vi "Change.vi"(0 "STEP in":refnum<class "STEP.lvclass">, 1 "Variables State":T3, 2 "SEQ":refnum<queue>, 3 "STEP State":T4, 4 "Current Sequence":T1, 5 "error in (no error)":errorcluster) -> (14 "STEP out":refnum<class "STEP.lvclass">, 15 "Variables State out":T3, 17 "STEP State out":T4, 19 "error out":errorcluster)   [LabVIEW 2014, in "SeqLoop.lvlib" / "STEP Classes.lvlib" / "STEP.lvclass"]
doc: "Gestiona el cambio de pasos en función del estado de la condición de avance, error y alarma."
uses:
  STEP.lvclass
  TypeDefs/STEP State.ctl
  APIs/Message Queue/Message Cluster.ctl
  TypeDefs/Variables State.ctl
  TypeDefs/Sequence.ctl
  TypeDefs/LogicParsedExpression.ctl
  STEP.lvclass/STEP.ctl
  APIs/Message Queue/Enqueue Message (Single).vi
  SeqLoop.lvlib
  APIs/Message Queue/WINFAS 2 Message Queue.lvlib
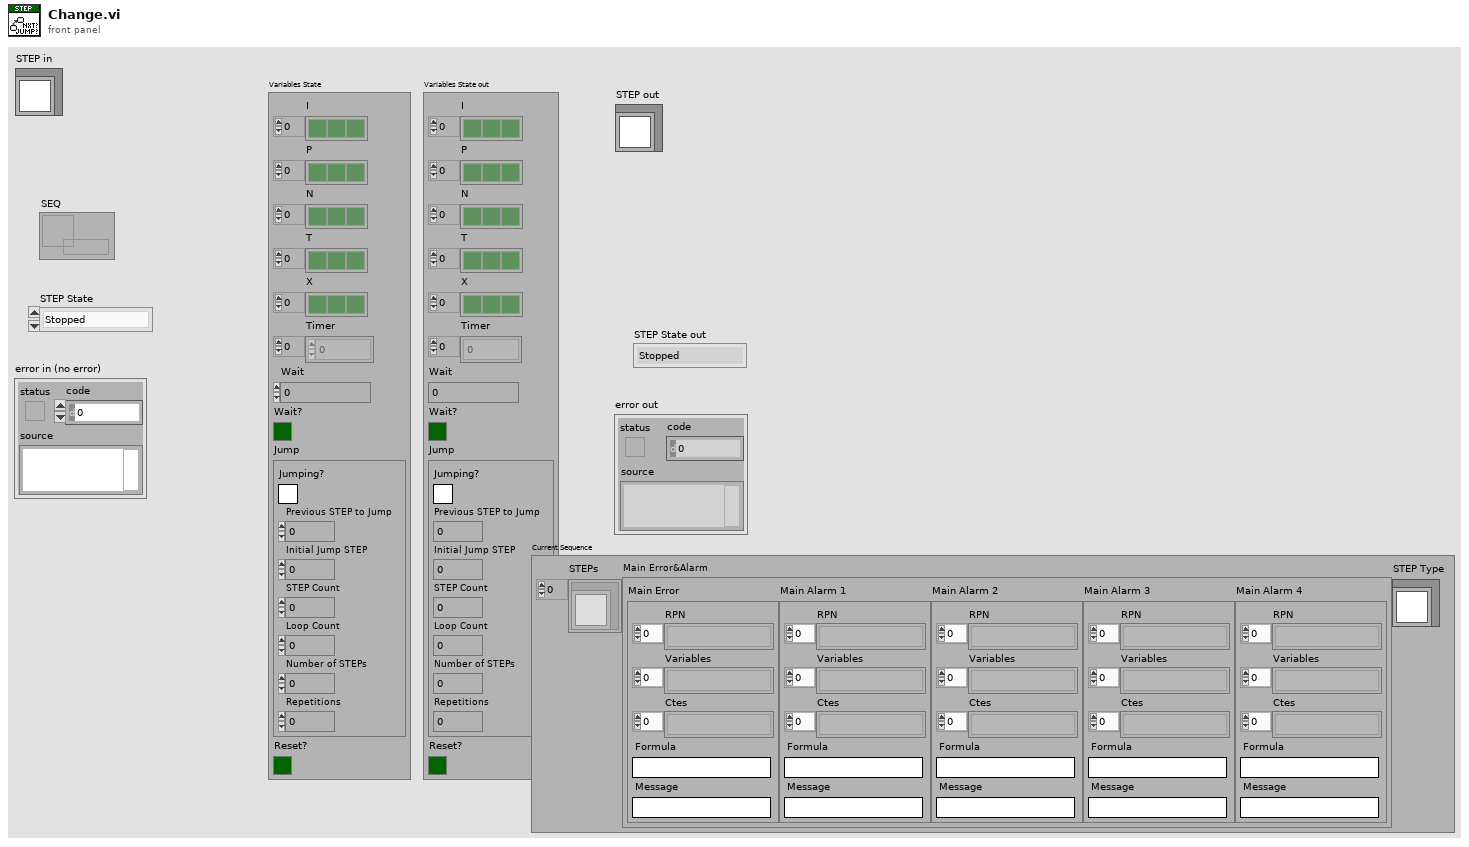
[diagram p1: front panel]
types:
  T1 = typedef "SeqLoop.lvlib/Sequence.ctl" = cluster{"STEPs":refnum<class "STEP.lvclass">[], "Main Error&Alarm":cluster{"Main Error":T2, "Main Alarm 1":T2, "Main Alarm 2":T2, "Main Alarm 3":T2, "Main Alarm 4":T2}, "STEP Type":refnum<class "STEP.lvclass">}
  T2 = typedef "SeqLoop.lvlib/LogicParsedExpression.ctl" = cluster{"RPN ":string[], "Variables":string[], "Ctes":string[], "Formula":string, "Message":string}
  T3 = typedef "SeqLoop.lvlib/Variables State.ctl" = cluster{"I":bool[], "P":bool[], "N":bool[], "T":bool[], "X":bool[], "Timer":u32[], "Wait":u32, "Wait?":bool, "Jump":cluster{"Jumping?":bool, "Previous STEP to Jump":u32, "Initial Jump STEP":u32, "STEP Count":u32, "Loop Count":u32, "Number of STEPs":u32, "Repetitions":u32}, "Reset?":bool}
  T4 = typedef "SeqLoop.lvlib/STEP State.ctl" = enum16{"Stopped", "First Call", "Idle...", "Advance OK", "Alarm", "Output Security", "Error"}
  T5 = cluster{"Jumping?":bool, "Previous STEP to Jump":u32, "Initial Jump STEP":u32, "STEP Count":u32, "Loop Count":u32, "Number of STEPs":u32, "Repetitions":u32}
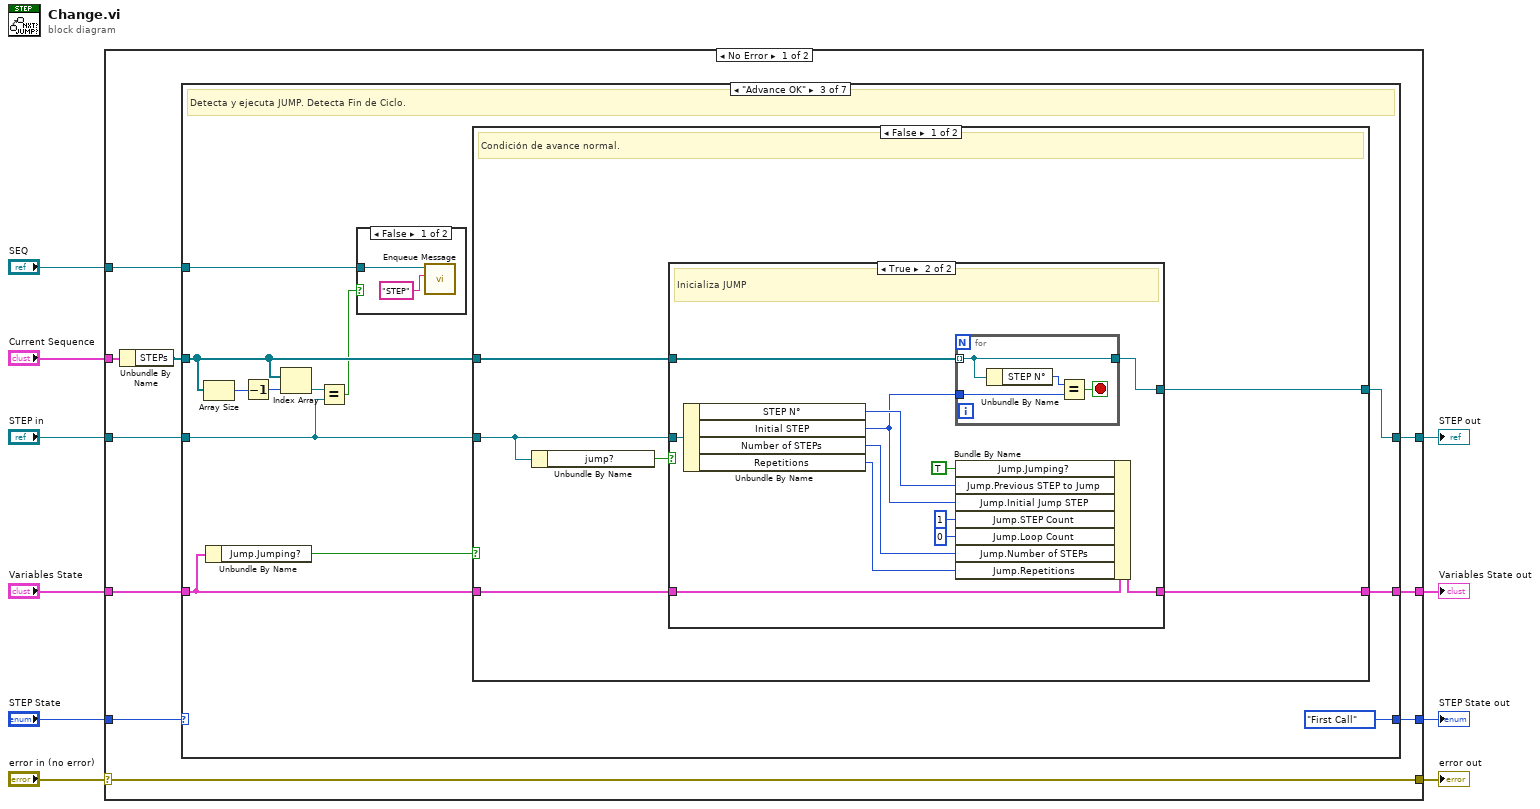
[diagram p0: block diagram]
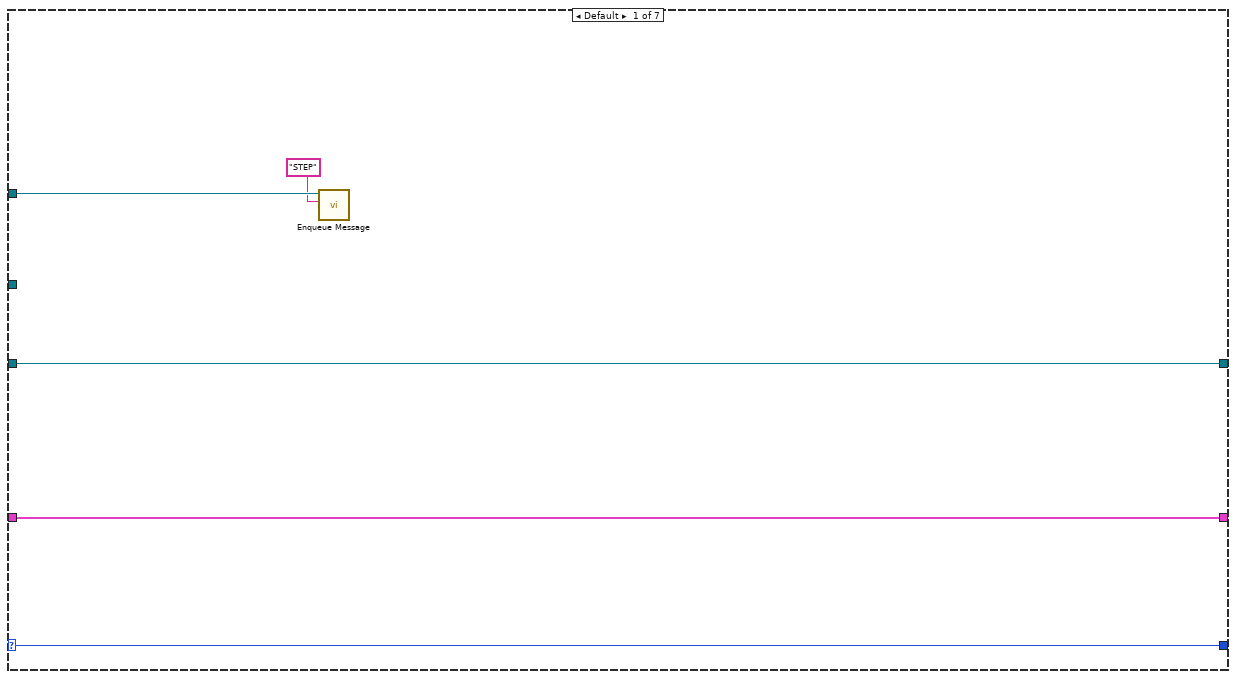
[diagram p2: hidden frame]
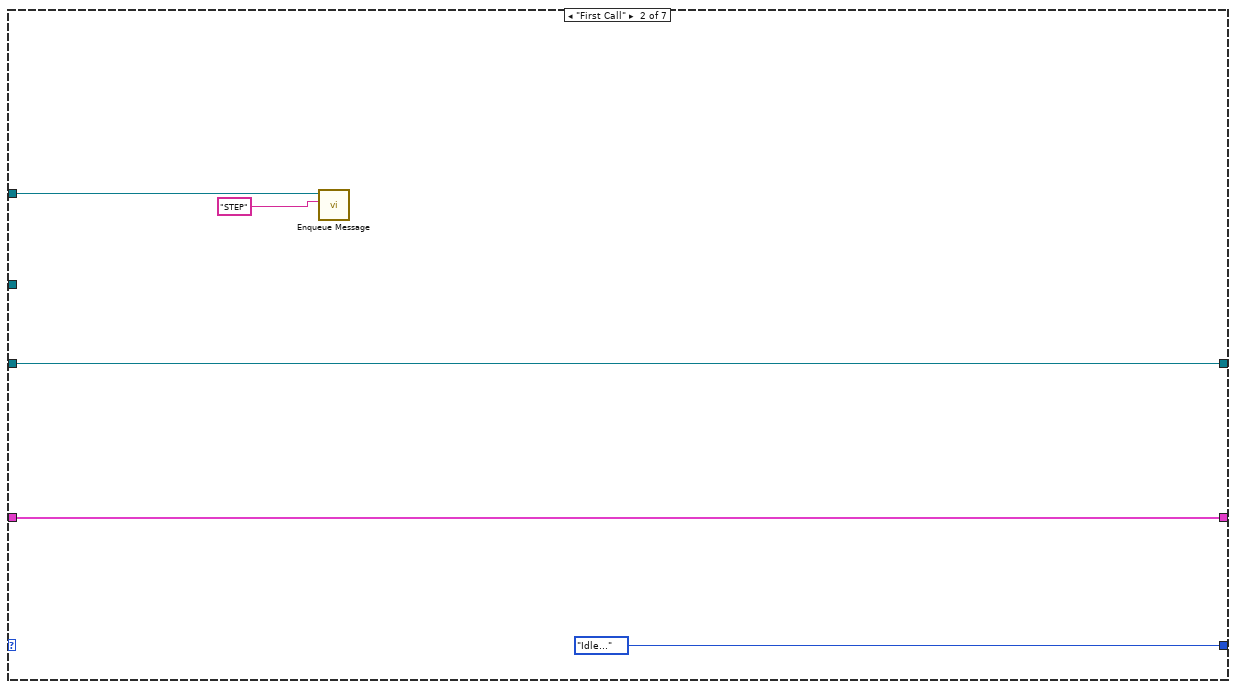
[diagram p3: hidden frame]
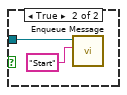
[diagram p4: hidden frame]
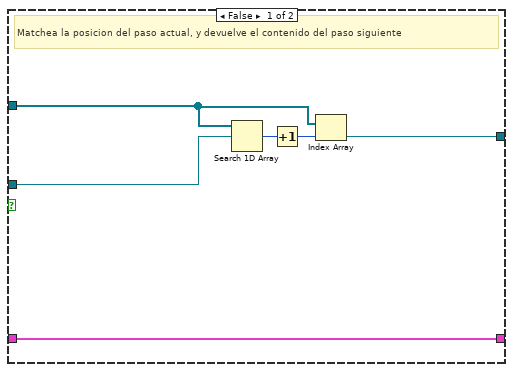
[diagram p5: hidden frame]
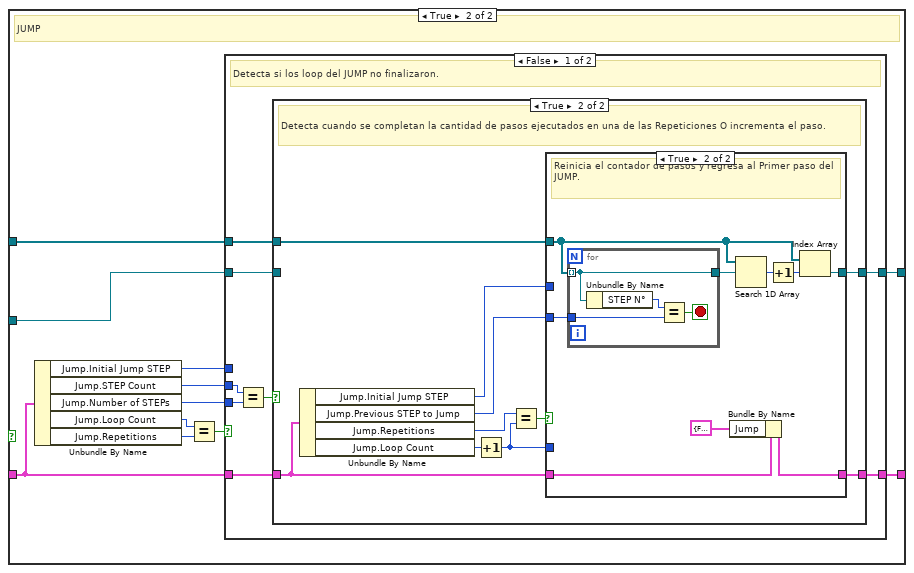
[diagram p6: hidden frame]
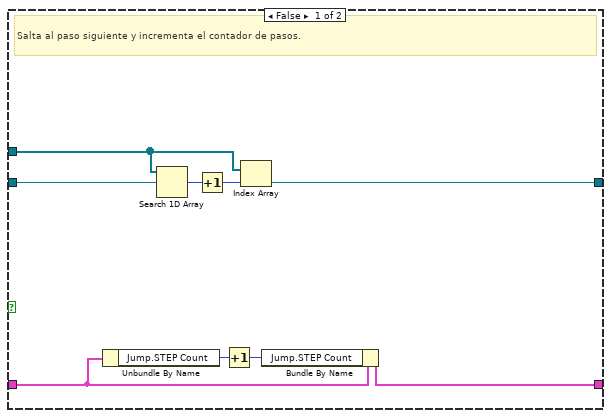
[diagram p7: hidden frame]
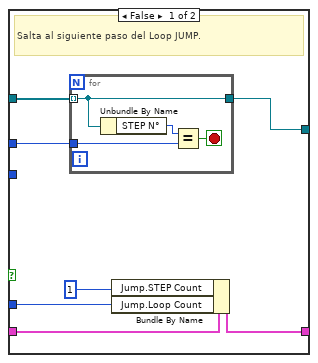
[diagram p8: hidden frame]
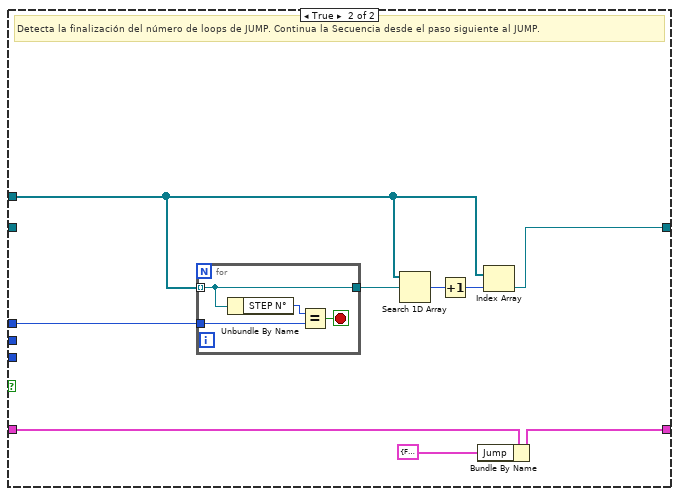
[diagram p9: hidden frame]
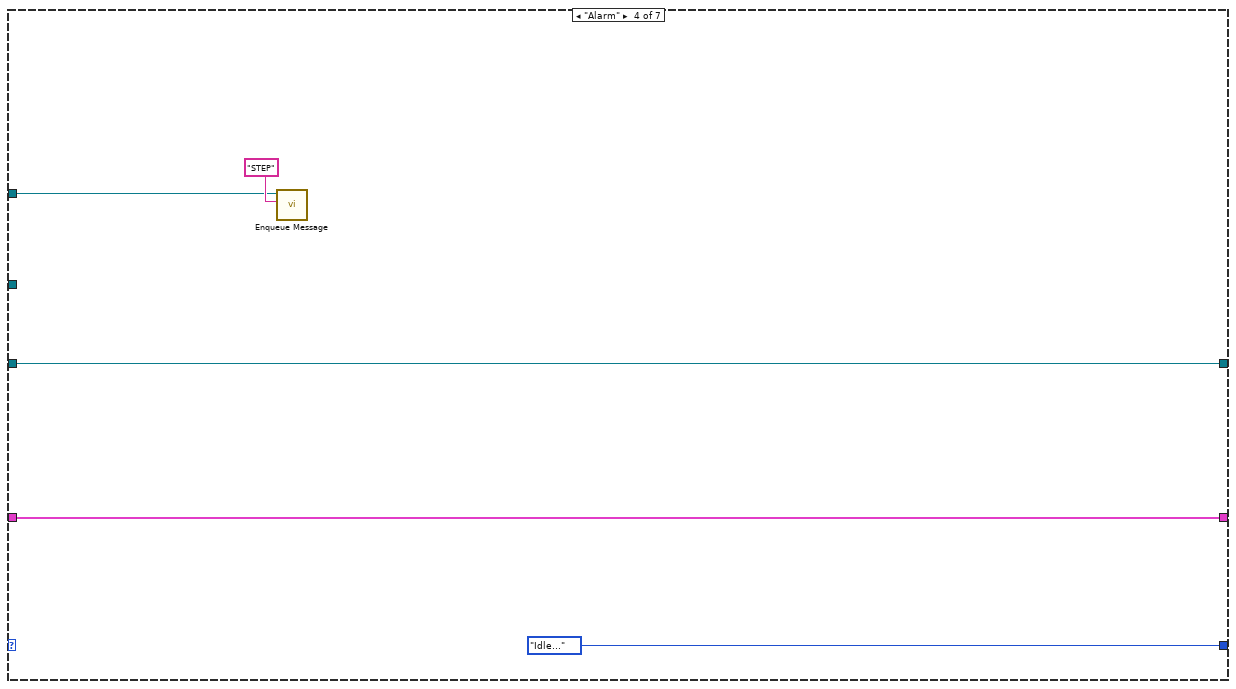
[diagram p10: hidden frame]
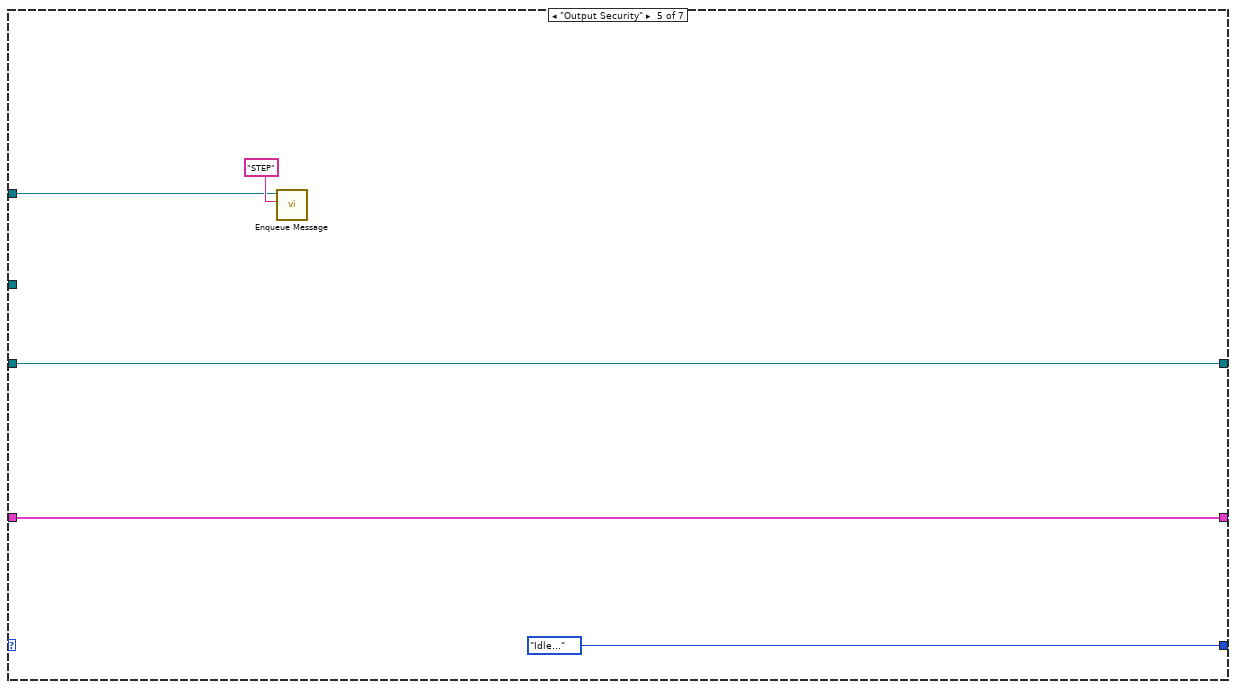
[diagram p11: hidden frame]
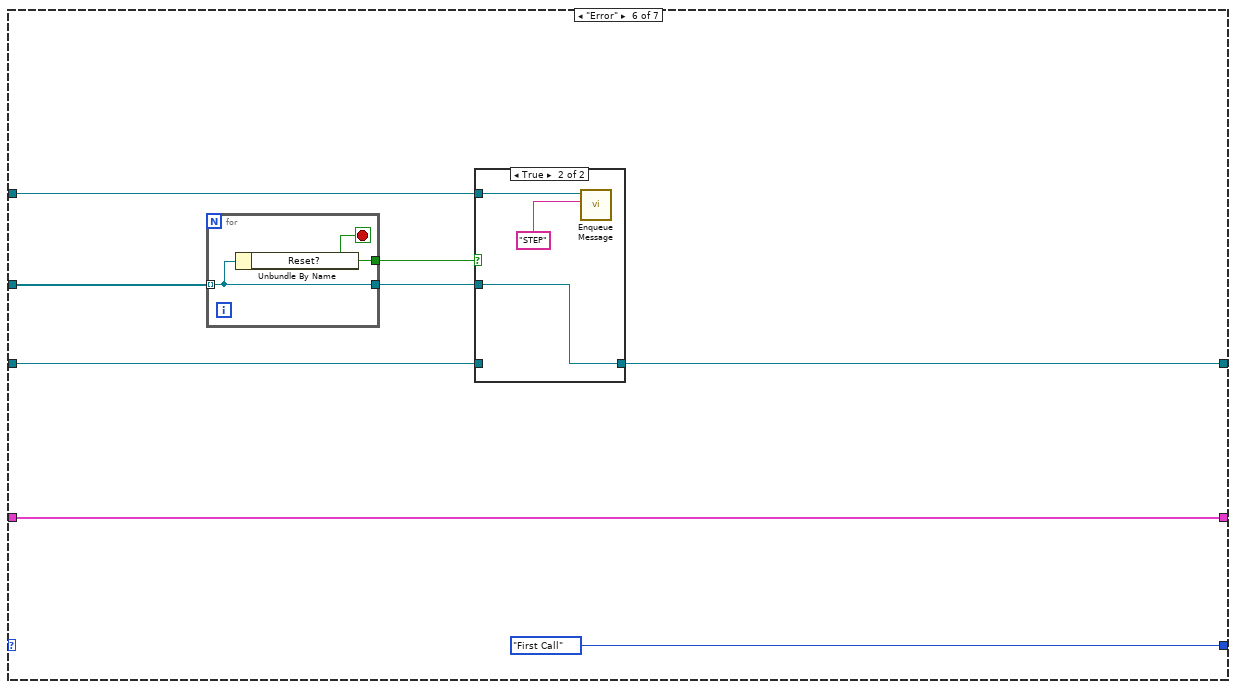
[diagram p12: hidden frame]
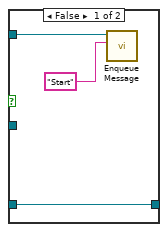
[diagram p13: hidden frame]
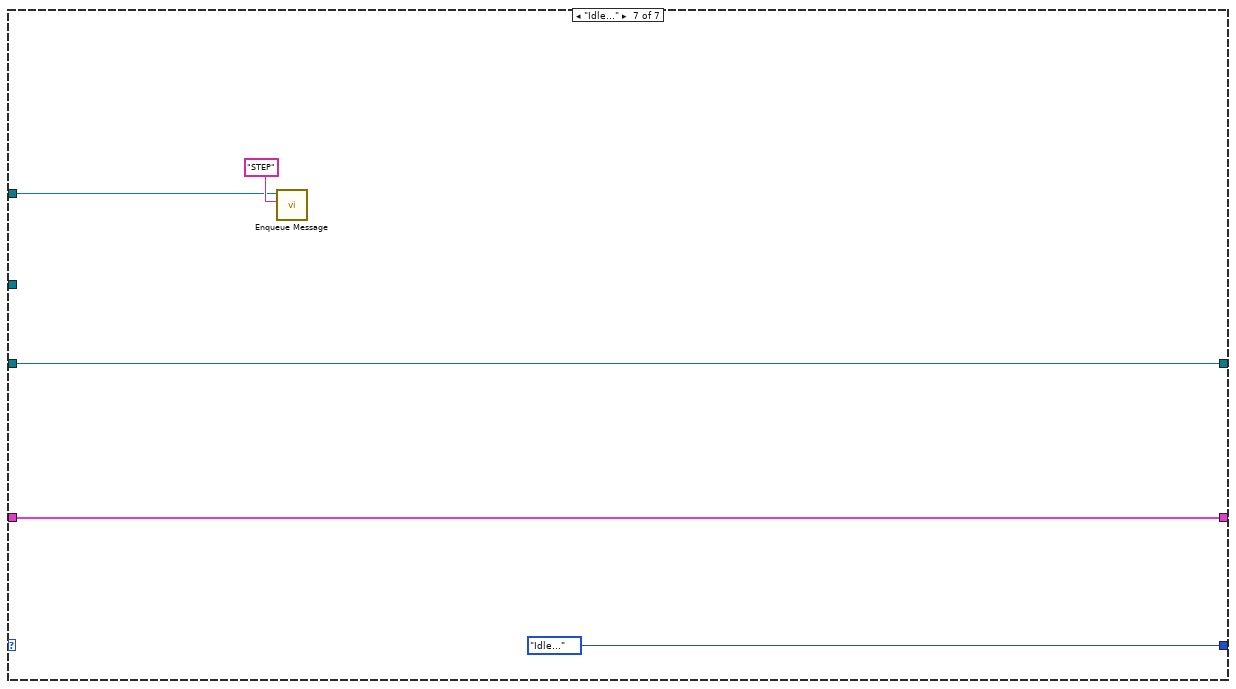
[diagram p14: hidden frame]
diagram:
  n1 = case shown="No Error" "error in (no error)" {
    selector: "error in (no error)" -> [w20 w184]
    tunnel: [w20 w184] -> w9
    tunnel: [w16 w183] -> w7
    tunnel: "STEP in" -> [w17 w183]
    tunnel: "STEP State" -> [w19 w182]
    tunnel: [w18 w182] -> w5
    tunnel: "Current Sequence" -> [w12 _]
    tunnel: "SEQ" -> [w15 _]
    tunnel: "Variables State" -> [w14 w181]
    tunnel: [w13 w181] -> w2
    frame No Error {
      n2 = Unbundle By Name(w12) -> ("STEPs"=w11:refnum<class "STEP.lvclass">[])
      n3 = case shown="\"Advance OK\"" w19 {
        selector: w19 -> [w24 _ _ _ _ _ _]
        tunnel: [w24 STEP_State."Idle..." ("STEP State") STEP_State."First Call" ("STEP State") STEP_State."Idle..." ("STEP State") STEP_State."Idle..." ("STEP State") STEP_State."First Call" ("STEP State") STEP_State."Idle..." ("STEP State")] -> w18
        tunnel: w11 -> [_ _ w36 _ _ w162 _]
        tunnel: w17 -> [w25 w30 w33 w153 w158 w164 w179]
        tunnel: [w25 w30 w41 w153 w158 w163 w179] -> w16
        tunnel: w15 -> [w23 w29 w40 w151 w156 w166 w177]
        tunnel: w14 -> [w21 w26 w39 w150 w155 w165 w176]
        tunnel: [w21 w26 w37 w150 w155 w165 w176] -> w13
        frame Default {
          n4 = call-poly "Enqueue Message.vi"("Message"="STEP", "Message Queue"=w23) -> ()  [unwired: 8 in, 2 out]
        }
        frame "First Call" {
          n5 = call-poly "Enqueue Message.vi"("Message"="STEP", "Message Queue"=w29) -> ()  [unwired: 8 in, 2 out]
        }
        frame "Advance OK" {
          # "Detecta y ejecuta JUMP. Detecta Fin de Ciclo."
          n6 = Array Size(array=w36) -> (size(s)=w35:i32)
          n7 = Unbundle By Name(w39) -> ("Jump.Jumping?"=w38:bool)
          n8 = Decrement(x=w35) -> (x-1=w34:i32)
          n9 = Index Array(array=w36, index=w34) -> (element=w32:refnum<class "STEP.lvclass">)
          n10 = Equal?(x=w32, y=w33) -> (x = y?=w31:bool)
          n11 = case shown="False" w31 {
            tunnel: w40 -> [w43 w45]
            frame False {
              n12 = call-poly "Enqueue Message.vi"("Message"="STEP", "Message Queue"=w43) -> ()  [unwired: 8 in, 2 out]
            }
            frame True {
              n13 = call-poly "Enqueue Message.vi"("Message"="Start", "Message Queue"=w45) -> ()  [unwired: 8 in, 2 out]
            }
          }
          n14 = case shown="False" w38 {
            tunnel: w36 -> [w52 w80]
            tunnel: [w50 w79] -> w41
            tunnel: w33 -> [w49 w76]
            tunnel: w39 -> [w48 w78]
            tunnel: [w47 w77] -> w37
            frame False {
              # "Condición de avance normal."
              n15 = Unbundle By Name(w49) -> ("jump?"=w51:bool)
              n16 = case shown="True" w51 {
                tunnel: w52 -> [w55 w70]
                tunnel: [w56 w69] -> w50
                tunnel: w49 -> [w54 w68]
                tunnel: w48 -> [w53 w67]
                tunnel: [w53 w61] -> w47
                frame False {
                  # "Matchea la posicion del paso actual, y devuelve el contenido del paso siguiente"
                  n17 = Search 1D Array(1D array=w55, element=w54) -> (index of element=w58:i32)  [unwired: 1 in]
                  n18 = Increment(x=w58) -> (x+1=w57:i32)
                  n19 = Index Array(array=w55, index=w57) -> (element=w56:refnum<class "STEP.lvclass">)
                }
                frame True {
                  # "Inicializa JUMP"
                  n20 = Unbundle By Name(w68) -> ("STEP N°"=w64:u32, "Initial STEP"=w59:u32, "Number of STEPs"=w65:u32, "Repetitions"=w66:u32)
                  n21 = for {
                    tunnel: w70 -> [w72] mode=indexing
                    tunnel: w59 -> [w73]
                    tunnel: [w72] -> w69
                    stop <- w71 stop-if-true
                    n22 = Unbundle By Name(w72) -> ("STEP N°"=w74:u32)
                    n23 = Equal?(x=w74, y=w73) -> (x = y?=w71:bool)
                  }
                  n24 = Bundle By Name(cluster=w67, "Jump.Jumping?"=TRUE, "Jump.Previous STEP to Jump"=w64, "Jump.Initial Jump STEP"=w59, "Jump.STEP Count"=u32 1, "Jump.Loop Count"=u32 0, "Jump.Number of STEPs"=w65, "Jump.Repetitions"=w66) -> (w61:T3)
                }
              }
            }
            frame True {
              # "JUMP"
              n25 = Unbundle By Name(w78) -> ("Jump.Initial Jump STEP"=w75:u32, "Jump.STEP Count"=w81:u32, "Jump.Number of STEPs"=w82:u32, "Jump.Loop Count"=w85:u32, "Jump.Repetitions"=w84:u32)
              n26 = Equal?(x=w85, y=w84) -> (x = y?=w83:bool)
              n27 = case shown="False" w83 {
                tunnel: w82 -> [w92 _]
                tunnel: w81 -> [w91 _]
                tunnel: w80 -> [w90 w141]
                tunnel: [w89 w142] -> w79
                tunnel: w78 -> [w88 w140]
                tunnel: [w87 w139] -> w77
                tunnel: w76 -> [w86 _]
                tunnel: w75 -> [_ w137]
                frame False {
                  # "Detecta si los loop del JUMP no finalizaron."
                  n28 = Equal?(x=w91, y=w92) -> (x = y?=w93:bool)
                  n29 = case shown="True" w93 {
                    tunnel: w90 -> [w96 w110]
                    tunnel: [w94 w111] -> w89
                    tunnel: w88 -> [w102 w106]
                    tunnel: [w101 w108] -> w87
                    tunnel: w86 -> [w95 _]
                    frame False {
                      # "Salta al paso siguiente y incrementa el contador de pasos."
                      n30 = Unbundle By Name(w102) -> ("Jump.STEP Count"=w100:u32)
                      n31 = Search 1D Array(1D array=w96, element=w95) -> (index of element=w98:i32)  [unwired: 1 in]
                      n32 = Increment(x=w98) -> (x+1=w97:i32)
                      n33 = Increment(x=w100) -> (x+1=w99:u32)
                      n34 = Index Array(array=w96, index=w97) -> (element=w94:refnum<class "STEP.lvclass">)
                      n35 = Bundle By Name(cluster=w102, "Jump.STEP Count"=w99) -> (w101:T3)
                    }
                    frame True {
                      # "Detecta cuando se completan la cantidad de pasos ejecutados en una de las Repeticiones O incrementa el paso."
                      n36 = Unbundle By Name(w106) -> ("Jump.Initial Jump STEP"=w103:u32, "Jump.Previous STEP to Jump"=w104:u32, "Jump.Repetitions"=w107:u32, "Jump.Loop Count"=w112:u32)
                      n37 = Increment(x=w112) -> (x+1=w105:u32)
                      n38 = Equal?(x=w107, y=w105) -> (x = y?=w109:bool)
                      n39 = case shown="True" w109 {
                        tunnel: [w117 w132] -> w111
                        tunnel: w110 -> [w119 w130]
                        tunnel: w103 -> [w118 _]
                        tunnel: w104 -> [_ w129]
                        tunnel: w106 -> [w114 w127]
                        tunnel: [w113 w126] -> w108
                        tunnel: w105 -> [w115 _]
                        frame False {
                          # "Salta al siguiente paso del Loop JUMP."
                          n40 = for {
                            tunnel: w119 -> [w121] mode=indexing
                            tunnel: w118 -> [w122]
                            tunnel: [w121] -> w117
                            stop <- w120 stop-if-true
                            n41 = Unbundle By Name(w121) -> ("STEP N°"=w123:u32)
                            n42 = Equal?(x=w123, y=w122) -> (x = y?=w120:bool)
                          }
                          n43 = Bundle By Name(cluster=w114, "Jump.STEP Count"=u32 1, "Jump.Loop Count"=w115) -> (w113:T3)
                        }
                        frame True {
                          # "Reinicia el contador de pasos y regresa al Primer paso del JUMP."
                          n44 = for {
                            tunnel: w130 -> [w134] mode=indexing
                            tunnel: w129 -> [w135]
                            tunnel: [w134] -> w131
                            stop <- w133 stop-if-true
                            n45 = Unbundle By Name(w134) -> ("STEP N°"=w136:u32)
                            n46 = Equal?(x=w136, y=w135) -> (x = y?=w133:bool)
                          }
                          n47 = Bundle By Name(cluster=w127, "Jump"=T5 {"Jumping?"=FALSE, "Previous STEP to Jump"=0, "Initial Jump STEP"=0, "STEP Count"=1, "Loop Count"=0, "Number of STEPs"=0, "Repetitions"=0}) -> (w126:T3)
                          n48 = Search 1D Array(1D array=w130, element=w131) -> (index of element=w125:i32)  [unwired: 1 in]
                          n49 = Increment(x=w125) -> (x+1=w124:i32)
                          n50 = Index Array(array=w130, index=w124) -> (element=w132:refnum<class "STEP.lvclass">)
                        }
                      }
                    }
                  }
                }
                frame True {
                  # "Detecta la finalización del número de loops de JUMP. Continua la Secuencia desde el paso siguiente al JUMP."
                  n51 = for {
                    tunnel: w141 -> [w147] mode=indexing
                    tunnel: w137 -> [w148]
                    tunnel: [w147] -> w143
                    stop <- w146 stop-if-true
                    n52 = Unbundle By Name(w147) -> ("STEP N°"=w149:u32)
                    n53 = Equal?(x=w149, y=w148) -> (x = y?=w146:bool)
                  }
                  n54 = Search 1D Array(1D array=w141, element=w143) -> (index of element=w145:i32)  [unwired: 1 in]
                  n55 = Increment(x=w145) -> (x+1=w144:i32)
                  n56 = Bundle By Name(cluster=w140, "Jump"=T5 {"Jumping?"=FALSE, "Previous STEP to Jump"=0, "Initial Jump STEP"=0, "STEP Count"=1, "Loop Count"=0, "Number of STEPs"=0, "Repetitions"=0}) -> (w139:T3)
                  n57 = Index Array(array=w141, index=w144) -> (element=w142:refnum<class "STEP.lvclass">)
                }
              }
            }
          }
        }
        frame "Alarm" {
          n58 = call-poly "Enqueue Message.vi"("Message"="STEP", "Message Queue"=w151) -> ()  [unwired: 8 in, 2 out]
        }
        frame "Output Security" {
          n59 = call-poly "Enqueue Message.vi"("Message"="STEP", "Message Queue"=w156) -> ()  [unwired: 8 in, 2 out]
        }
        frame "Error" {
          n60 = for {
            tunnel: w162 -> [w169] mode=indexing
            tunnel: [w169] -> w161
            tunnel: [w168] -> w160
            stop <- w168 stop-if-true
            n61 = Unbundle By Name(w169) -> ("Reset?"=w168:bool)
          }
          n62 = case shown="True" w160 {
            tunnel: w166 -> [w171 w174]
            tunnel: w164 -> [w170 _]
            tunnel: w161 -> [_ w173]
            tunnel: [w170 w173] -> w163
            frame False {
              n63 = call-poly "Enqueue Message.vi"("Message"="Start", "Message Queue"=w171) -> ()  [unwired: 8 in, 2 out]
            }
            frame True {
              n64 = call-poly "Enqueue Message.vi"("Message"="STEP", "Message Queue"=w174) -> ()  [unwired: 8 in, 2 out]
            }
          }
        }
        frame "Idle..." {
          n65 = call-poly "Enqueue Message.vi"("Message"="STEP", "Message Queue"=w177) -> ()  [unwired: 8 in, 2 out]
        }
      }
    }
    frame Error {
    }
  }
  "error out" <- w9
  "STEP out" <- w7
  "STEP State out" <- w5
  "Variables State out" <- w2
